vi "Get Element.vi"(8 "element":string, 9 "category":string, 11 "Datastore.Dictionaries in":refnum<class "Datastore.Dictionaries.lvclass">) -> (0 "element dup":string, 1 "category dup":string, 2 "Value":variant, 3 "Datastore.Dictionaries":refnum<class "Datastore.Dictionaries.lvclass">, 4 "found?":bool)   [LabVIEW 2021, in "Bananas.lvlib" / "Datastore.Dictionaries.lvclass"]
uses:
  Datastore.Dictionaries.lvclass
  Datastore.Dictionaries.lvclass/Datastore.Dictionaries.ctl
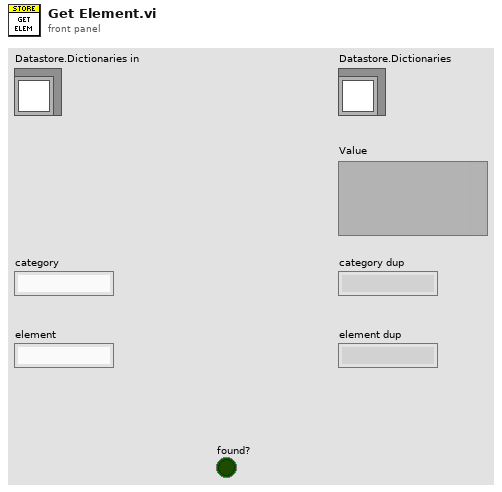
[diagram p1: front panel]
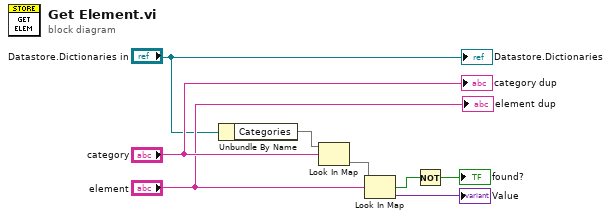
[diagram p0: block diagram]
diagram:
  n1 = Unbundle By Name("Datastore.Dictionaries in") -> ("Categories"=w8:map{string, map{string, variant}})
  n2 = Look In Map(map=w8, key="category") -> (value=w7:map{string, variant})  [unwired: 1 in, 1 out]
  n3 = Look In Map(map=w7, key="element") -> (key not found?=w5:bool, value=→"Value":variant)  [unwired: 1 in]
  n4 = Not(x=w5) -> (.not. x?=→"found?":bool)
  "category dup" <- "category"
  "element dup" <- "element"
  "Datastore.Dictionaries" <- "Datastore.Dictionaries in"
